vi "ILAB_ViStatus.vi"(4 "name":string) -> (0 "errorOut":string, 1 "status":i32)   [LabVIEW 2009]
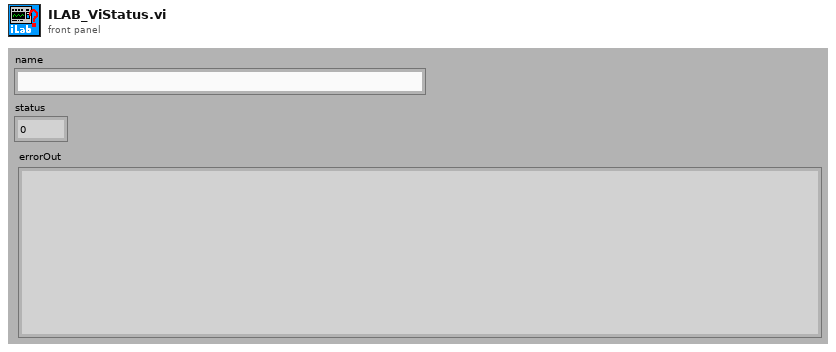
[diagram p1: front panel]
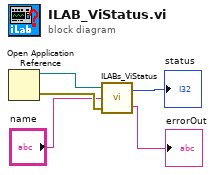
[diagram p0: block diagram]
diagram:
  n1 = Open Application Reference() -> (0:w3:errorcluster, 3:w4:refnum<vi>)  [unwired: 1 in, 3 out]
  n2 = call "ILABs_ViStatus.vi"("errorIn"=w3, "name"="name", "appReference"=w4) -> ("errorOut"=→"errorOut":string, "status"=→"status":i32)
